vi "Launch Numeric Keypad Dialog Box.vi"(4 "Auto-stop? (T)":bool=TRUE, 8 "error in (no error)":errorcluster, 9 "Parameter Name":string, 10 "Reply Transport":refnum<class "ITransport.lvclass">, 11 "Dialog Launcher In":refnum<class "IViewable.lvclass">) -> (0 "error out":errorcluster, 3 "Dialog Launcher Out":refnum<class "IViewable.lvclass">)   [LabVIEW 2017, in "NumericKeypadDialogBox.lvlib" / "NumericKeypadDialogBox.lvclass"]
uses:
  NumericKeypadDialogBox.lvclass
  gpm_packages/@cs/mva-viewable/Source/IViewable/IViewable/IViewable.lvclass
  gpm_packages/@cs/transport/Source/ITransport/ITransport.lvclass
  C:/Git/mva-framework/Source/IDialogBox/IDialogBox/IDialogBox.lvclass
  NumericKeypadDialogBox.lvclass/NumericKeypadDialogBox.ctl
  IDialogBox/IDialogBox/IDialogBox.lvclass
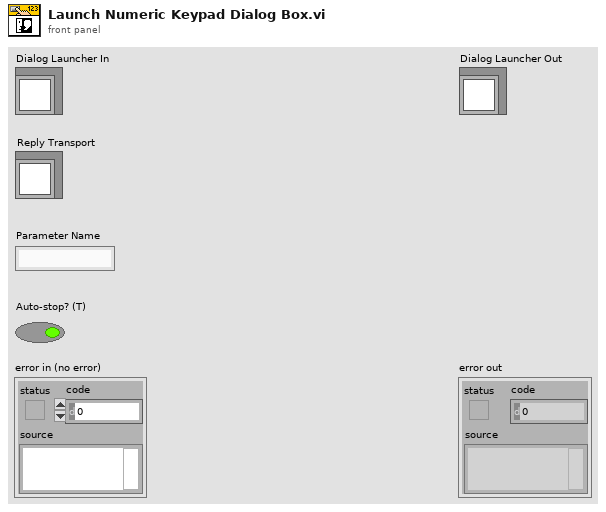
[diagram p1: front panel]
types:
  T1 = enum32{"Invalid", "Default", "Floating", "Floating/Auto-Hide", "Modal"}
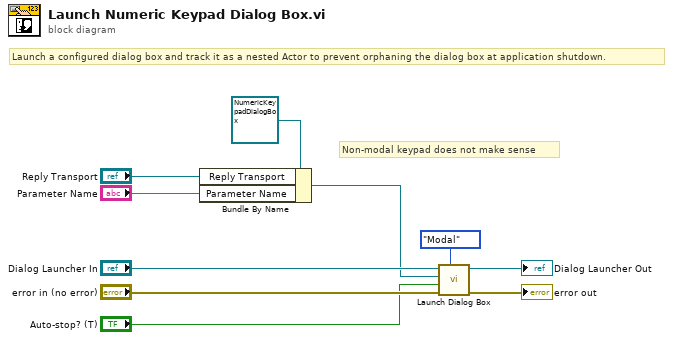
[diagram p0: block diagram]
diagram:
  # "Non-modal keypad does not make sense"
  # "Launch a configured dialog box and track it as a nested Actor to prevent orphaning the dialog box at application shutdown."
  n1 = Bundle By Name(cluster=refnum<class "NumericKeypadDialogBox.lvclass"> refnum ("OneButtonDialogBox in"), "Reply Transport"="Reply Transport", "Parameter Name"="Parameter Name") -> (w2:refnum<class "NumericKeypadDialogBox.lvclass">)
  n2 = call "Launch Dialog Box.vi"("FP Window:Behavior (Floating)"=T1."Modal" ("FP Window:Behavior"), "error in (no error)"="error in (no error)", "Auto-stop? (T)"="Auto-stop? (T)", "DialogBox"=w2, "DialogBox Launcher"="Dialog Launcher In") -> ("error out"=→"error out":errorcluster, "DialogBox Launcher Out"=→"Dialog Launcher Out":refnum<class "IViewable.lvclass">)  [unwired: 4 in, 1 out]
